vi "String_2_Number_array.vi"(1 "Input String":string[](array[string])) -> (0 "Values":dbl[](array[numeric]))   [LabVIEW 2010]
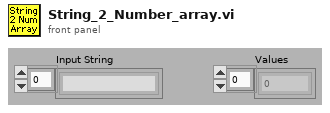
[diagram p1: front panel]
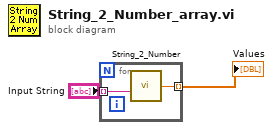
[diagram p0: block diagram]
diagram:
  n1 = for {
    tunnel: "Input String" -> [w4] mode=indexing
    tunnel: [w3] -> w2 mode=indexing
    n2 = call "String_2_Number.vi"("Value"=w4) -> ("Numeric"=w3:dbl)
  }
  "Values" <- w2
